vi "shutdown.vi"(8 "error in":errorcluster, 9 "state":T1, 10 "Boiler Controls":T3 {"Fuel Control Valve Position (% Open)" scale=0.0..100.0}, 11 "Boiler Simulation Controls":T2 {"Flame Sensor Value (%)" scale=0.0..100.0}) -> (0 "error out":errorcluster, 3 "state out":T1)   [LabVIEW 2015]
uses:
  controls/state.ctl
panel:
  # "On"
  # "Off"
  # "Closed"
  # "Open"
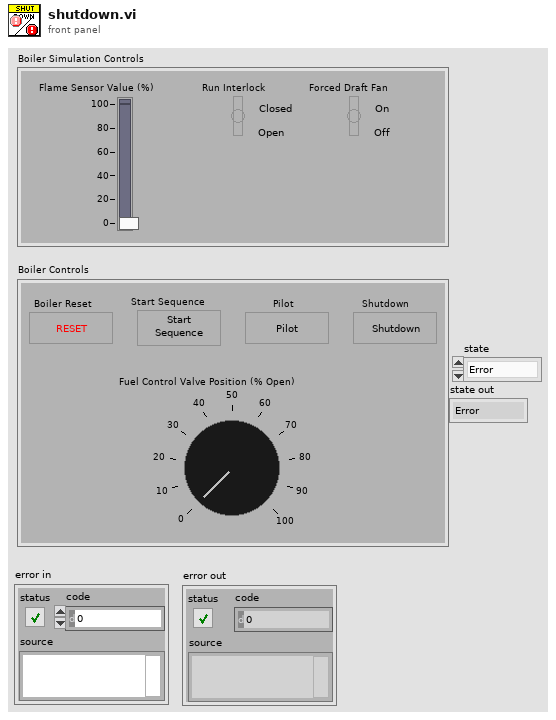
[diagram p1: front panel]
types:
  T1 = typedef "state.ctl" = enum16{"Error", "Exit", "Reset lockout", "Ignition", "Pre Purge Continue", "Pre Purge", "Wait", "Ready", "Initialize", "Purge", "Shutdown", "Run", "Start", "Prove Pilot"}
  T2 = cluster{"Flame Sensor Value (%)":dbl, "Run Interlock":bool, "Forced Draft Fan":bool}
  T3 = cluster{"Shutdown":bool, "Pilot Button":bool, "Start Sequence":bool, "Boiler Reset":bool, "Fuel Control Valve Position (% Open)":dbl}
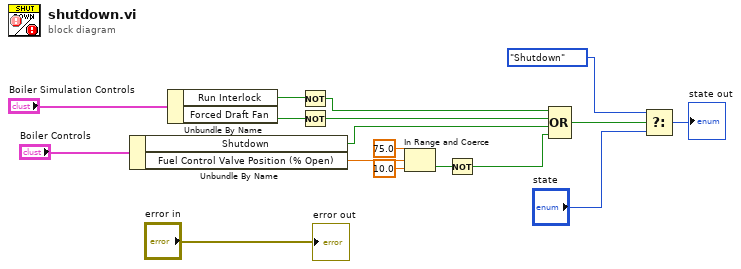
[diagram p0: block diagram]
diagram:
  n1 = Unbundle By Name("Boiler Controls") -> ("Shutdown"=w16:bool, "Fuel Control Valve Position (% Open)"=w10:dbl)
  n2 = Unbundle By Name("Boiler Simulation Controls") -> ("Run Interlock"=w2:bool, "Forced Draft Fan"=w14:bool)
  n3 = Not(x=w2) -> (.not. x?=w1:bool)
  n4 = Not(x=w14) -> (.not. x?=w17:bool)
  n5 = In Range and Coerce(upper limit=75.0, x=w10, lower limit=10.0) -> (In Range?=w13:bool)  [unwired: 1 out]
  n6 = Not(x=w13) -> (.not. x?=w15:bool)
  n7 = Compound Arithmetic op=OR(w1, w17, w16, w15) -> (w6:bool)
  n8 = Select(t=state."Shutdown" ("state"), s=w6, f="state") -> (s? t:f=→"state out":T1)
  "error out" <- "error in"
